vi "Get Receive Event.vi"(8 "error in":errorcluster, 11 "TPCANHandle in":T2=81 items=["PCAN_NONEBUS"=0, "PCAN_USBBUS1"=81, "PCAN_USBBUS2"=82, "PCAN_USBBUS3"=83, "PCAN_USBBUS4"=84, "PCAN_USBBUS5"=85, "PCAN_USBBUS6"=86, "PCAN_USBBUS7"=87, "PCAN_USBBUS8"=88, "PCAN_USBBUS9"=1289, "PCAN_USBBUS10"=1290, "PCAN_USBBUS11"=1291, "PCAN_USBBUS12"=1292, "PCAN_USBBUS13"=1293, "PCAN_USBBUS14"=1294, "PCAN_USBBUS15"=1295, "PCAN_USBBUS16"=1296]) -> (0 "error out":errorcluster, 1 "Filedescriptor fd (Linux)":i32, 2 "Event Handle (Win)":u64, 3 "TPCANHandle out":T2=81 items=["PCAN_NONEBUS"=0, "PCAN_USBBUS1"=81, "PCAN_USBBUS2"=82, "PCAN_USBBUS3"=83, "PCAN_USBBUS4"=84, "PCAN_USBBUS5"=85, "PCAN_USBBUS6"=86, "PCAN_USBBUS7"=87, "PCAN_USBBUS8"=88, "PCAN_USBBUS9"=1289, "PCAN_USBBUS10"=1290, "PCAN_USBBUS11"=1291, "PCAN_USBBUS12"=1292, "PCAN_USBBUS13"=1293, "PCAN_USBBUS14"=1294, "PCAN_USBBUS15"=1295, "PCAN_USBBUS16"=1296], 5 "TPCANStatus":T1 items=["PCAN_ERROR_OK"=0, "PCAN_ERROR_XMTFULL"=1, "PCAN_ERROR_OVERRUN"=2, "PCAN_ERROR_BUSLIGHT"=4, "PCAN_ERROR_BUSHEAVY"=8, "PCAN_ERROR_BUSPASSIVE"=262144, "PCAN_ERROR_BUSOFF"=16, "PCAN_ERROR_QRCVEMPTY"=32, "PCAN_ERROR_QOVERRUN"=64, "PCAN_ERROR_QXMTFULL"=128, "PCAN_ERROR_REGTEST"=256, "PCAN_ERROR_NODRIVER"=512, "PCAN_ERROR_HWINUSE"=1024, "PCAN_ERROR_NETINUSE"=2048, "PCAN_ERROR_ILLHW"=5120, "PCAN_ERROR_ILLNET"=6144, "PCAN_ERROR_ILLCLIENT"=7168, "PCAN_ERROR_RESOURCE"=8192, "PCAN_ERROR_ILLPARAMTYPE"=16384, "PCAN_ERROR_ILLPARAMVAL"=32768, "PCAN_ERROR_UNKNOWN"=65536, "PCAN_ERROR_ILLDATA"=131072, "PCAN_ERROR_ILLMODE"=524288, "PCAN_ERROR_CAUTION"=33554432, "PCAN_ERROR_INITIALIZE"=67108864, "PCAN_ERROR_ILLOPERATION"=134217728])   [LabVIEW 2020, in "PCANBasic.lvlib"]
doc: "This parameter is used to identify the state of use of a PCAN-Channel by returning a flag value. For example, a\nconnection is only possible when a PCAN-Channel is available, which means:\nIt is valid: The PCAN-Channel is one of the listed in the section “Supported by” below.\nIt is connectable: The PCAN-Channel is not initialized, or it is currently used by a PCAN-View application."
uses:
  PCANBasic.lvlib
  TPCANParameter.ctl
  peak/PCANBasic64.dll
  TPCANHandle.ctl
  TPCANStatus.ctl
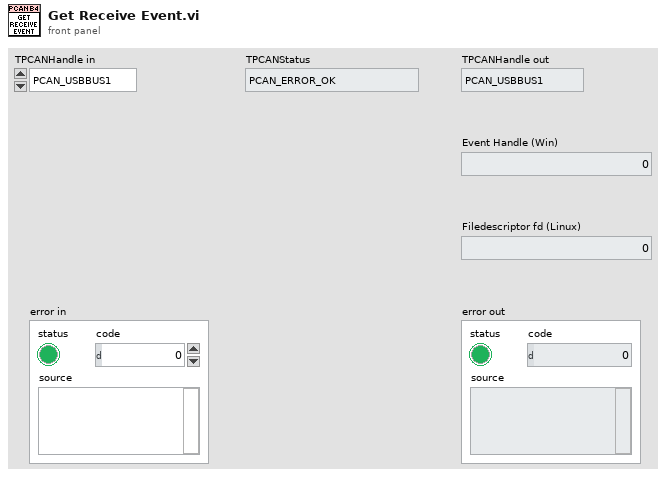
[diagram p1: front panel]
types:
  T1 = typedef "PCANBasic.lvlib/TPCANStatus.ctl" = u32
  T2 = typedef "PCANBasic.lvlib/TPCANHandle.ctl" = u16
  T3 = typedef "PCANBasic.lvlib/TPCANParameter.ctl" = enum8{"Unknown", "PCAN_DEVICE_ID", "PCAN_5VOLTS_POWER", "PCAN_RECEIVE_EVENT", "PCAN_MESSAGE_FILTER", "PCAN_API_VERSION", "PCAN_CHANNEL_VERSION", "PCAN_BUSOFF_AUTORESET", "PCAN_LISTEN_ONLY", "PCAN_LOG_LOCATION", "PCAN_LOG_STATUS", "PCAN_LOG_CONFIGURE", "PCAN_LOG_TEXT", "PCAN_CHANNEL_CONDITION", "PCAN_HARDWARE_NAME", "PCAN_RECEIVE_STATUS", "PCAN_CONTROLLER_NUMBER", "PCAN_TRACE_LOCATION", "PCAN_TRACE_STATUS", "PCAN_TRACE_SIZE", "PCAN_TRACE_CONFIGURE", "PCAN_CHANNEL_IDENTIFYING", "PCAN_CHANNEL_FEATURES", "PCAN_BITRATE_ADAPTING", "PCAN_BITRATE_INFO", "PCAN_BITRATE_INFO_FD", "PCAN_BUSSPEED_NOMINAL", "PCAN_BUSSPEED_DATA", "PCAN_IP_ADDRESS", "PCAN_LAN_SERVICE_STATUS", "PCAN_ALLOW_STATUS_FRAMES", "PCAN_ALLOW_RTR_FRAMES", "PCAN_ALLOW_ERROR_FRAMES", "PCAN_INTERFRAME_DELAY", "PCAN_ACCEPTANCE_FILTER_11BIT", "PCAN_ACCEPTANCE_FILTER_29BIT", "PCAN_IO_DIGITAL_CONFIGURATION", "PCAN_IO_DIGITAL_VALUE", "PCAN_IO_DIGITAL_SET", "PCAN_IO_DIGITAL_CLEAR", "PCAN_IO_ANALOG_VALUE", "PCAN_FIRMWARE_VERSION", "PCAN_ATTACHED_CHANNELS_COUNT", "PCAN_ATTACHED_CHANNELS", "PCAN_ALLOW_ECHO_FRAMES", "PCAN_DEVICE_PART_NUMBER", "PCAN_HARD_RESET_STATUS", "PCAN_LAN_CHANNEL_DIRECTION", "PCAN_DEVICE_GUID"}
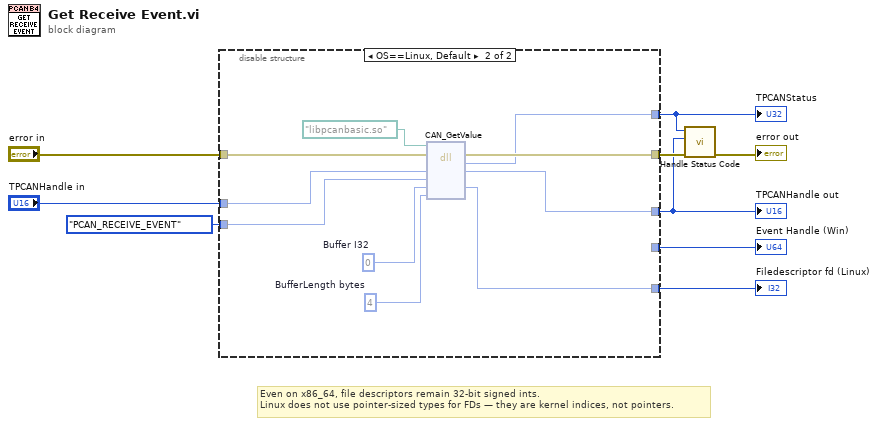
[diagram p0: block diagram]
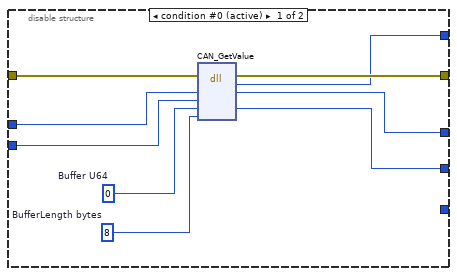
[diagram p2: hidden frame]
diagram:
  # "Even on x86_64, file descriptors remain 32-bit signed ints.\nLinux does not use pointer-sized types for FDs — they are kernel indices, not pointers."
  n1 = disable-structure shown="OS==Linux, Default" {
    disable-tunnel: "TPCANHandle in" -> [w18 w21]
    disable-tunnel: "error in" -> [w17 w28]
    disable-tunnel: [w16 w27] -> w7
    disable-tunnel: TPCANParameter."PCAN_RECEIVE_EVENT" ("TPCANParameter") -> [w15 w26]
    disable-tunnel: [w12 w22] -> w2
    disable-tunnel: [w11 w20] -> w1
    disable-tunnel: [w10 _] -> w4
    disable-tunnel: [_ w24] -> w3
    frame condition #0 (active) {
      w13 = u32 8  # BufferLength bytes
      w14 = u64 0  # Buffer U64
      n2 = dll-call lib="D:/git/PCAN-Basic-LabVIEW/source/peak/PCANBasic*.dll" fn="CAN_GetValue"(error in=w17, "Channel"=w18, "TPCANParameter"=w15, "Buffer"=w14, "BufferLength"=w13) -> (error out=w16:errorcluster, "TPCANStatus"=w12:u32, "Channel"=w11:u16, "Buffer"=w10:u64)  [unwired: 4 in, 1 out]
    }
    frame condition #1 {
      w23 = u32 4  # BufferLength bytes
      w25 = 0  # Buffer I32
      n3 = dll-call lib="?" fn="CAN_GetValue"(path in=path "libpcanbasic.so", error in=w28, "Channel"=w21, "TPCANParameter"=w26, "Buffer"=w25, "BufferLength"=w23) -> (error out=w27:errorcluster, "TPCANStatus"=w22:u32, "Channel"=w20:u16, "Buffer"=w24:i32)  [unwired: 3 in, 1 out]
    }
  }
  "TPCANHandle out" <- w1
  "TPCANStatus" <- w2
  "Event Handle (Win)" <- w4
  "Filedescriptor fd (Linux)" <- w3
  n4 = call "Handle Status Code.vi"("error in"=w7, "TPCANHandle"=w1, "TPCANStatus"=w2) -> ("error out"=→"error out":errorcluster)  [unwired: 8 in]
